vi "Calculate Playback Position.vi"(11 "Status":T1={"VI"={"error"={"status"=FALSE, "code"=0, "source"=""}, "isExiting?"=FALSE}, "UserLoggedIn?"=FALSE, "Processors"={"Video A"=refnum, "Video B"=refnum, "Averaging Type"=enum."Normal Average", "Roughness Processor"=refnum}, "Playback"={"FPS"=10.0, "Playing?"=FALSE, "Playable?"=FALSE, "Image A"=refnum, "Image B"=refnum}, "Mouse Position A"=0.0, "Mouse Position B"=0.0}) -> (1 "Position":dbl, 3 "Status Out":T1={"VI"={"error"={"status"=FALSE, "code"=0, "source"=""}, "isExiting?"=FALSE}, "UserLoggedIn?"=FALSE, "Processors"={"Video A"=refnum, "Video B"=refnum, "Averaging Type"=enum."Normal Average", "Roughness Processor"=refnum}, "Playback"={"FPS"=10.0, "Playing?"=FALSE, "Playable?"=FALSE, "Image A"=refnum, "Image B"=refnum}, "Mouse Position A"=0.0, "Mouse Position B"=0.0})   [LabVIEW 2018]
uses:
  Status STYP.ctl
  Video Processor/Video Processor.lvclass
  Roughness Averager/Roughness Averager.lvclass
  <vilib>/vision/Image Controls.llb/IMAQ Image.ctl
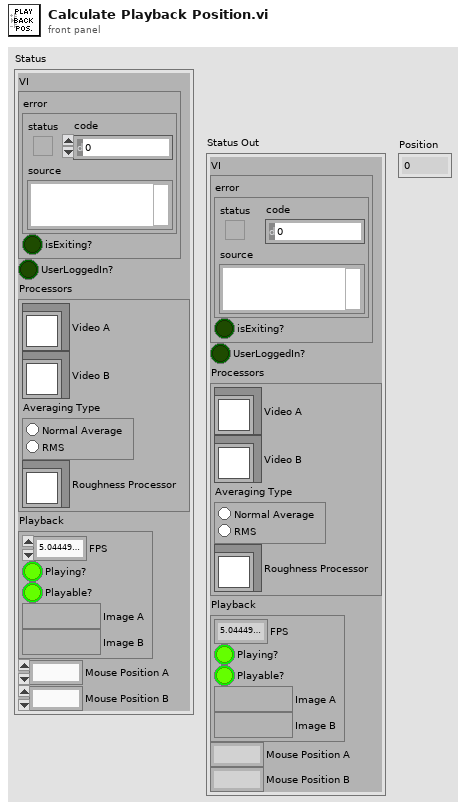
[diagram p1: front panel]
types:
  T1 = typedef "Status STYP.ctl" = cluster{"VI":cluster{"error":errorcluster, "isExiting?":bool}, "UserLoggedIn?":bool, "Processors":cluster{"Video A":refnum<class "Video Processor.lvclass">, "Video B":refnum<class "Video Processor.lvclass">, "Averaging Type":enum32{"Normal Average", "RMS"}, "Roughness Processor":refnum<class "Roughness Averager.lvclass">}, "Playback":cluster{"FPS":dbl, "Playing?":bool, "Playable?":bool, "Image A":T2, "Image B":T2}, "Mouse Position A":dbl, "Mouse Position B":dbl}
  T2 = typedef "IMAQ Image.ctl" = refnum<image>
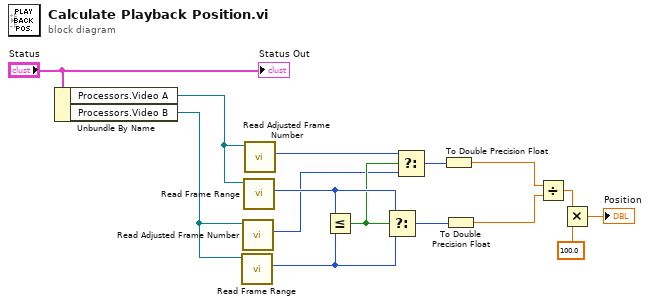
[diagram p0: block diagram]
diagram:
  n1 = Unbundle By Name("Status") -> ("Processors.Video A"=w7:refnum<class "Video Processor.lvclass">, "Processors.Video B"=w8:refnum<class "Video Processor.lvclass">)
  n2 = call-dynamic "Read Frame Range.vi"("Video File in"=w8) -> ("Number of Frames"=w5:u32)  [unwired: 8 in, 2 out]
  n3 = call-dynamic "Read Adjusted Frame Number.vi"("Video File in"=w8) -> ("Frame Number"=w2:u32)  [unwired: 8 in, 2 out]
  n4 = call-dynamic "Read Frame Range.vi"("Video File in"=w7) -> ("Number of Frames"=w6:u32)  [unwired: 8 in, 2 out]
  n5 = call-dynamic "Read Adjusted Frame Number.vi"("Video File in"=w7) -> ("Frame Number"=w3:u32)  [unwired: 8 in, 2 out]
  n6 = Less Or Equal?(x=w6, y=w5) -> (x <= y?=w4:bool)
  n7 = Select(t=w6, s=w4, f=w5) -> (s? t:f=w15:u32)
  n8 = Select(t=w3, s=w4, f=w2) -> (s? t:f=w1:u32)
  n9 = To Double Precision Float(number=w1) -> (double precision float=w13:dbl)
  n10 = To Double Precision Float(number=w15) -> (double precision float=w14:dbl)
  n11 = Divide(x=w13, y=w14) -> (x/y=w12:dbl)
  n12 = Multiply(x=w12, y=100.0) -> (x*y=→"Position":dbl)
  "Status Out" <- "Status"
